vi "is_finished.vi"(7 "duration":dbl[unit], 8 "error in (no error)":errorcluster, 9 "current image time stamp":timestamp, 10 "start image time stamp":timestamp, 11 "MG090623BinningImageAssembler in":refnum<class "ImageAssemblerMG090623Binning.lvclass">) -> (0 "error out":errorcluster, 2 "finished?":bool, 3 "MG090623BinningImageAssembler out":refnum<class "ImageAssemblerMG090623Binning.lvclass">)   [LabVIEW 2010, in "ImageAssemblerMG090623Binning.lvclass"]
uses:
  ImageAssemblerMG090623Binning.lvclass
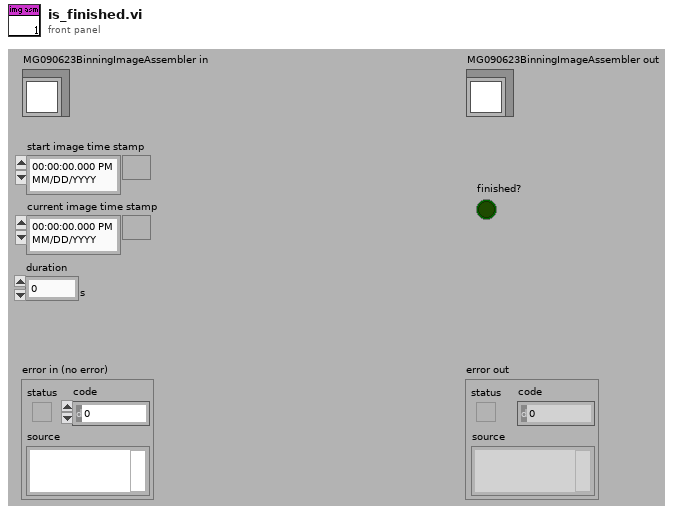
[diagram p1: front panel]
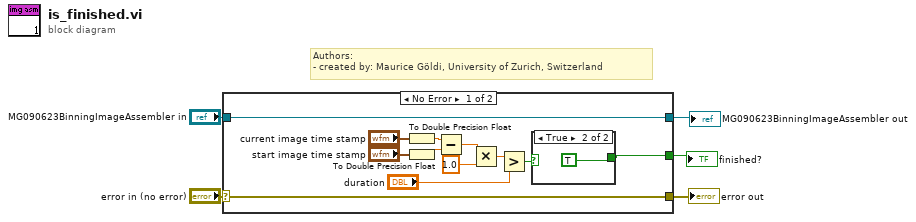
[diagram p0: block diagram]
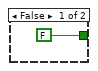
[diagram p2: hidden frame]
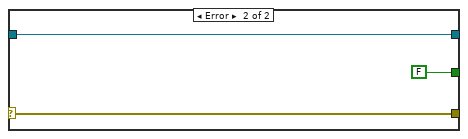
[diagram p3: hidden frame]
diagram:
  # "Authors: \n- created by: Maurice Göldi, University of Zurich, Switzerland"
  n1 = case shown="No Error" "error in (no error)" {
    selector: "error in (no error)" -> [w16 w22]
    tunnel: [w16 w22] -> w4
    tunnel: [w17 w21] -> w2
    tunnel: "MG090623BinningImageAssembler in" -> [w17 w21]
    tunnel: [w15 FALSE] -> w1
    frame No Error {
      n2 = To Double Precision Float(number="current image time stamp") -> (double precision float=w9:dbl)
      n3 = To Double Precision Float(number="start image time stamp") -> (double precision float=w8:dbl)
      n4 = Subtract(x=w9, y=w8) -> (x-y=w11:dbl)
      n5 = Multiply(x=w11, y=dbl[unit] 1.0) -> (x*y=w12:dbl[unit])
      n6 = Greater?(x=w12, y="duration") -> (0:w14:bool)
      n7 = case shown="True" w14 {
        tunnel: [FALSE TRUE] -> w15
        frame False {
        }
        frame True {
        }
      }
    }
    frame Error {
    }
  }
  "error out" <- w4
  "MG090623BinningImageAssembler out" <- w2
  "finished?" <- w1
